vi "读取消息.vi"(8 "error in (no error)":errorcluster caption="错误输入（无错误）", 11 "消息类输入":refnum<class "消息类.lvclass">) -> (0 "error out":errorcluster caption="错误输出", 2 "消息":string, 3 "消息类输出":refnum<class "消息类.lvclass">)   [LabVIEW 2016, in "消息类.lvclass"]
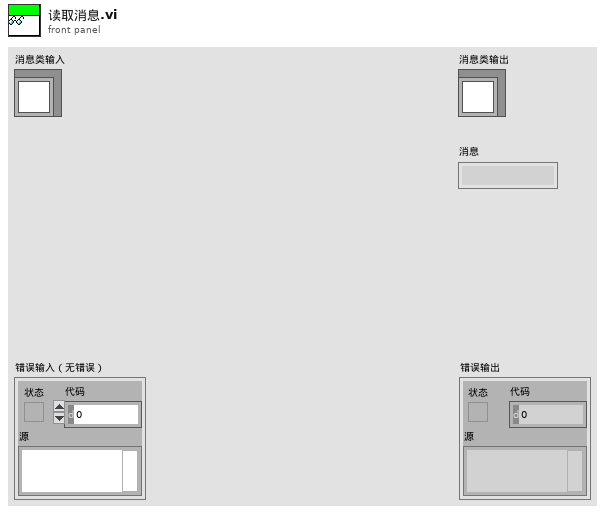
[diagram p1: front panel]
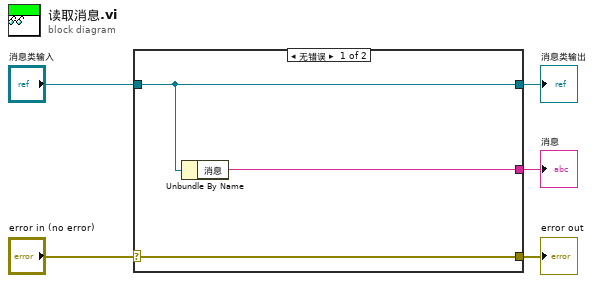
[diagram p0: block diagram]
diagram:
  n1 = case shown="无错误" "error in (no error)" {
    selector: "error in (no error)" -> [w8 w9]
    tunnel: [w8 w9] -> w4
    tunnel: [w7 w10] -> w2
    tunnel: "消息类输入" -> [w7 w10]
    tunnel: [w6 _] -> w1
    frame No Error {
      n2 = Unbundle By Name(w7) -> ("消息"=w6:string)
    }
    frame Error {
    }
  }
  "error out" <- w4
  "消息类输出" <- w2
  "消息" <- w1
